vi "World Point To Local.vi"(9 "Rotation [deg]":sgl, 10 "Sprite Center":refnum<class "Vector 2D.lvclass">, 11 "World Point":refnum<class "Vector 2D.lvclass">) -> (3 "Local Point":refnum<class "Vector 2D.lvclass">)   [LabVIEW 2021]
uses:
  Re-use Libraries/Vector 2D/Vector 2D.lvclass
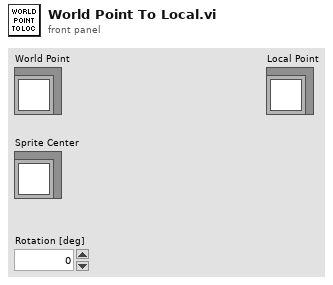
[diagram p1: front panel]
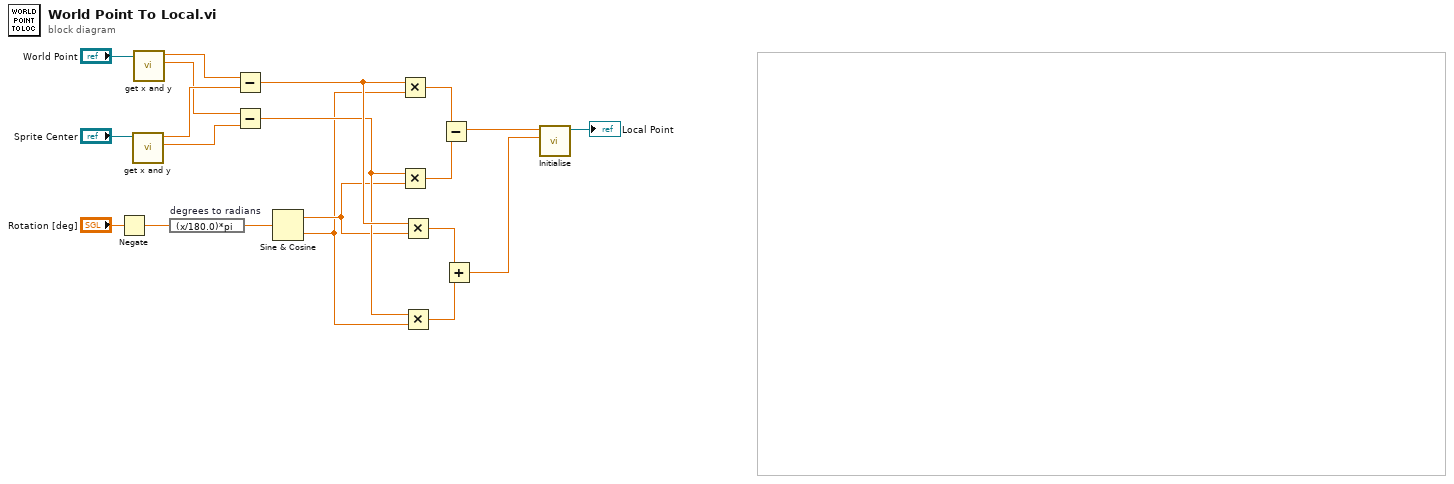
[diagram p0: block diagram]
diagram:
  n1 = Negate(x="Rotation [deg]") -> (-x=w12:sgl)
  n2 = call "get x and y.vi"("Vector 2D in"="Sprite Center") -> ("y"=w15:sgl, "x"=w17:sgl)  [unwired: 9 in]
  n3 = call "get x and y.vi"("Vector 2D in"="World Point") -> ("y"=w16:sgl, "x"=w18:sgl)  [unwired: 9 in]
  n4 = expression code="(x/180.0)*pi" "degrees to radians"(w12) -> (w14:sgl)
  n5 = Subtract(x=w18, y=w17) -> (x-y=w7:sgl)
  n6 = Subtract(x=w16, y=w15) -> (x-y=w6:sgl)
  n7 = Sine & Cosine(0:w14) -> (1:w5:sgl, 2:w4:sgl)
  n8 = Multiply(x=w7, y=w4) -> (x*y=w11:sgl)
  n9 = Multiply(x=w6, y=w5) -> (x*y=w10:sgl)
  n10 = Multiply(x=w7, y=w5) -> (x*y=w8:sgl)
  n11 = Multiply(x=w6, y=w4) -> (x*y=w9:sgl)
  n12 = Subtract(x=w11, y=w10) -> (x-y=w3:sgl)
  n13 = Add(x=w8, y=w9) -> (x+y=w2:sgl)
  n14 = call "Initialise.vi"("y"=w2, "x"=w3) -> ("Vector 2D out"=→"Local Point":refnum<class "Vector 2D.lvclass">)  [unwired: 9 in]
